vi "Set Cell Alignment.vi"(1 "Vertical alignment":T1, 4 "Horizontal alignment":T2, 5 "Text Rotation":i32 min=0 max=180 step=1, 6 "error in (no error)":errorcluster, 7 "End Cell Address":string, 8 "Wrap Text":bool, 9 "Start Cell Address":string, 10 "Report Ref In":T3) -> (0 "error out":errorcluster, 3 "Report Ref Out":T3)   [LabVIEW 2026, in "XCel Report Engine.lvlib"]
uses:
  XCel Report Engine.lvlib
  Controls/Report Ref.ctl
  C:/Users/m.santucci/Documents/ChatGPT/LV_REPORT_ENGINE/.net/src/XCelReportEngine/bin/Release/net48/XCelReportEngine.dll
  .net/src/XCelReportEngine/bin/Release/net48/XCelReportEngine.dll
  Controls/Horizontal alignment.ctl
  Controls/Vertical alignment.ctl
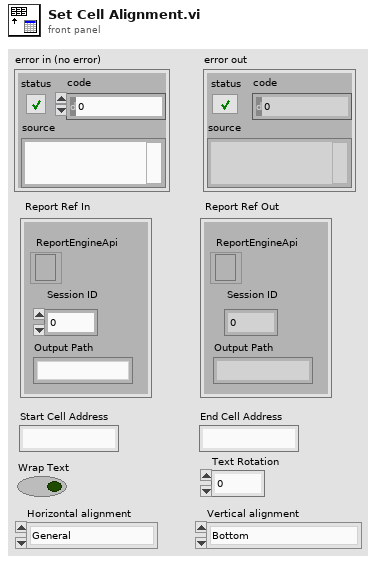
[diagram p1: front panel]
types:
  T1 = typedef "XCel Report Engine.lvlib/Vertical alignment.ctl" = enum16{"Bottom", "Center", "Top", "Justify", "Distributed"}
  T2 = typedef "XCel Report Engine.lvlib/Horizontal alignment.ctl" = enum16{"General", "Left", "Center", "Right", "Fill", "Justify", "CenterContinuous", "Distributed"}
  T3 = typedef "XCel Report Engine.lvlib/Report Ref.ctl" = cluster{"Session ID":i32, "Output Path":string, "ReportEngineApi":refnum<k24>}
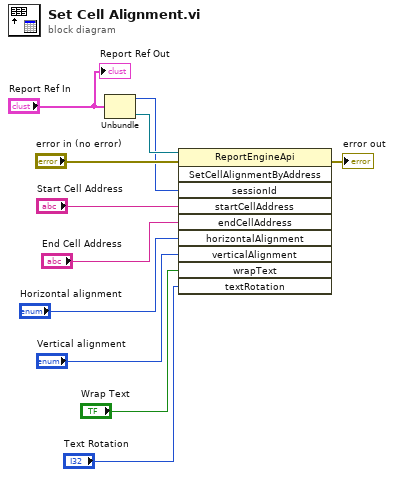
[diagram p0: block diagram]
diagram:
  n1 = Unbundle("Report Ref In") -> ("Session ID"=w7:i32, "ReportEngineApi"=w10:refnum<k24>)  [unwired: 1 out]
  n2 = invoke class="ReportEngineApi" method="SetCellAlignmentByAddress"(reference=w10, error in="error in (no error)", "sessionId"=w7, "startCellAddress"="Start Cell Address", "endCellAddress"="End Cell Address", "horizontalAlignment"="Horizontal alignment", "verticalAlignment"="Vertical alignment", "wrapText"="Wrap Text", "textRotation"="Text Rotation") -> (error out=→"error out":errorcluster)  [unwired: 1 in, 9 out]
  "Report Ref Out" <- "Report Ref In"
